vi "Determine Next Regulation Generation Level.vi"(8 "error in (no error)":errorcluster, 10 "current generation level":dbl, 11 "regulation settings":T1) -> (0 "error out":errorcluster, 3 "next generation level":dbl)   [LabVIEW 2021]
uses:
  controls/regulation target.ctl
  controls/regulation target value units.ctl
  controls/regulation settings.ctl
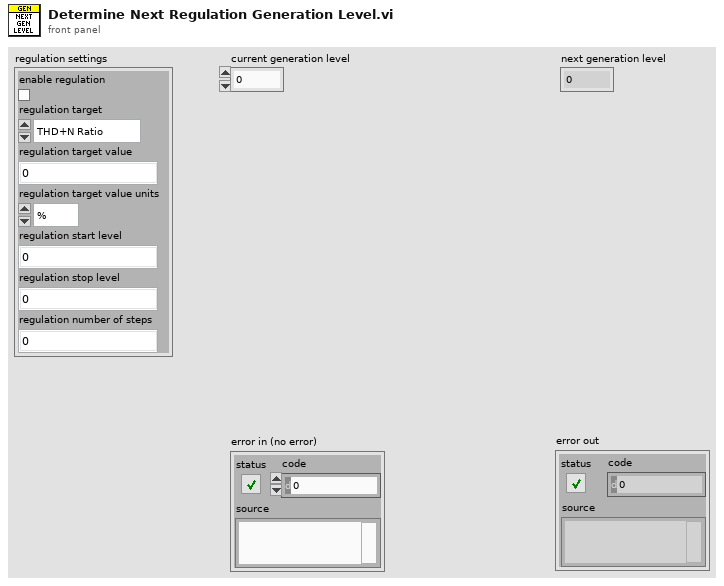
[diagram p1: front panel]
types:
  T1 = typedef "regulation settings.ctl" = cluster{"enable regulation":bool, "regulation target":T2, "regulation target value":dbl, "regulation target value units":T3, "regulation start level":dbl, "regulation stop level":dbl, "regulation number of steps":u32}
  T2 = typedef "regulation target.ctl" = enum32{"THD+N Ratio", "Output Power"}
  T3 = typedef "regulation target value units.ctl" = enum32{"%", "W"}
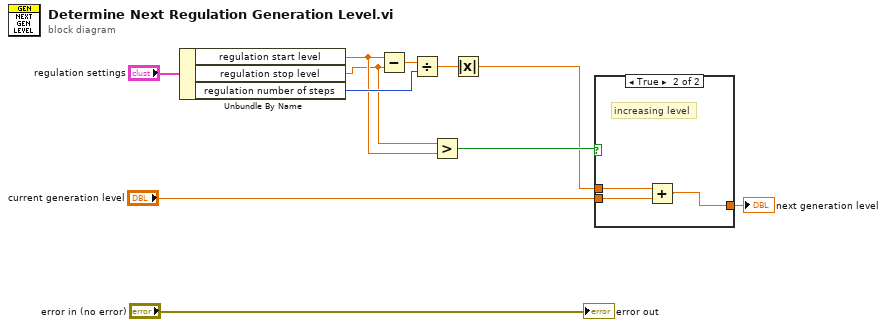
[diagram p0: block diagram]
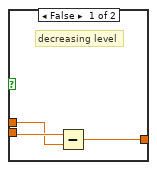
[diagram p2: hidden frame]
diagram:
  n1 = Unbundle By Name("regulation settings") -> ("regulation start level"=w5:dbl, "regulation stop level"=w4:dbl, "regulation number of steps"=w8:u32)
  n2 = Subtract(x=w5, y=w4) -> (x-y=w9:dbl)
  n3 = Divide(x=w9, y=w8) -> (x/y=w6:dbl)
  n4 = Greater?(x=w4, y=w5) -> (0:w3:bool)
  n5 = Absolute Value(x=w6) -> (abs(x)=w1:dbl)
  n6 = case shown="True" w3 {
    tunnel: "current generation level" -> [w14 w17]
    tunnel: w1 -> [w13 w16]
    tunnel: [w12 w15] -> w2
    frame False {
      # "decreasing level"
      n7 = Subtract(x=w14, y=w13) -> (x-y=w12:dbl)
    }
    frame True {
      # "increasing level"
      n8 = Add(x=w16, y=w17) -> (x+y=w15:dbl)
    }
  }
  "next generation level" <- w2
  "error out" <- "error in (no error)"
